vi "delete PID from engine.vi"(8 "error in (no error)":errorcluster, 9 "PID Loop in":T1, 10 "engine configuration in":refnum<class "engine configuration.lvclass">, 11 "Tagbus PID Module configuration in":refnum<class "PID Module configuration.lvclass">) -> (0 "error out":errorcluster, 1 "index":i32, 2 "engine configuration out":refnum<class "engine configuration.lvclass">, 3 "Tagbus PID Module configuration out":refnum<class "PID Module configuration.lvclass">)   [LabVIEW 2013, in "PID Module editor node.lvclass"]
uses:
  PID Module editor node.lvclass
  module/configuration/PID Module configuration.lvclass
  <vilib>/NI/Configuration Framework/serializable configuration/NISE_CEF_serializable configuration.lvclass
  <vilib>/NI/Module Execution Interface/Engine Configuration/engine configuration.lvclass
  PID array element.ctl
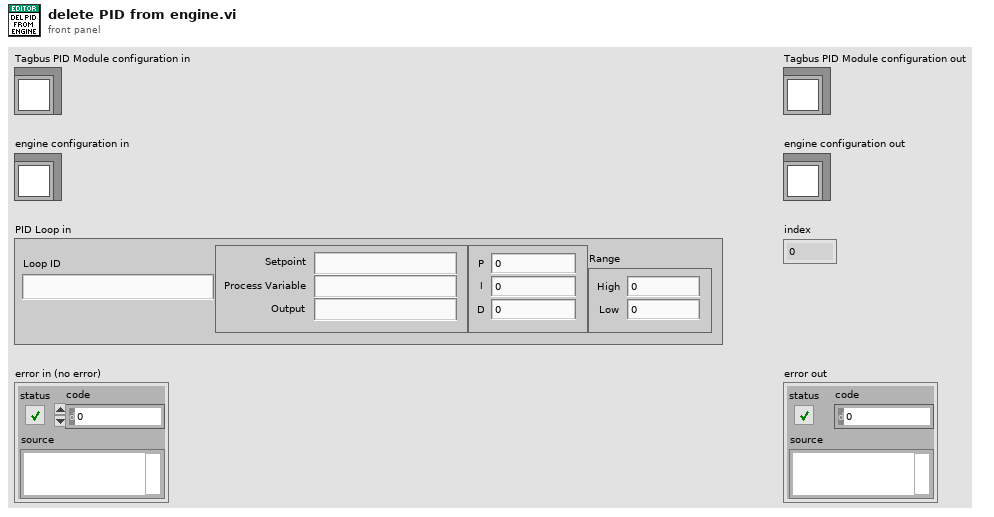
[diagram p1: front panel]
types:
  T1 = typedef "PID Module editor node.lvclass/PID array element.ctl" = cluster{"Loop ID":string, "Tags":cluster{"Setpoint":string, "Process Variable":string, "Output":string}, "Gains":cluster{"P":dbl, "I":dbl, "D":dbl}, "Range":cluster{"High":dbl, "Low":dbl}}
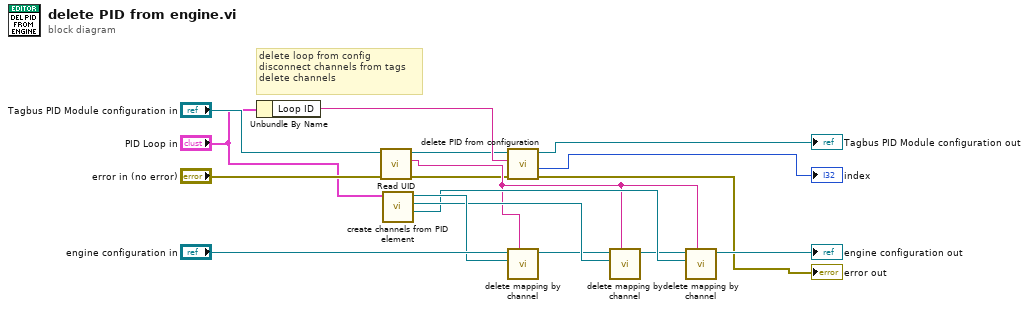
[diagram p0: block diagram]
diagram:
  # "delete loop from config\ndisconnect channels from tags\ndelete channels"
  n1 = Unbundle By Name("PID Loop in") -> ("Loop ID"=w16:string)
  n2 = call <vilib>:"Read UID.vi"("error in"="error in (no error)", "configuration in"="Tagbus PID Module configuration in") -> ("error out"=w2:errorcluster, "instance id"=w7:string, "configuration out"=w15:refnum<class "PID Module configuration.lvclass">)  [unwired: 7 in]
  n3 = call "create channels from PID element.vi"("line item in"="PID Loop in") -> ("Output Channel Out"=w8:refnum<class "TBM channel.lvclass">, "Process Variable Channel Out"=w9:refnum<class "TBM channel.lvclass">, "Setpoint Channel Out"=w10:refnum<class "TBM channel.lvclass">)  [unwired: 8 in]
  n4 = call "delete PID from configuration.vi"("error in"=w2, "PID Loop ID In"=w16, "Tagbus PID Module configuration in"=w15) -> ("error out"=→"error out":errorcluster, "index"=→"index":i32, "Tagbus PID Module configuration out"=→"Tagbus PID Module configuration out":refnum<class "PID Module configuration.lvclass">)  [unwired: 5 in, 1 out]
  n5 = call <vilib>:"delete mapping by channel.vi"("owner ID"=w7, "channel"=w10, "engine configuration in"="engine configuration in") -> ("engine configuration out"=w6:refnum<class "engine configuration.lvclass">)  [unwired: 7 in, 1 out]
  n6 = call <vilib>:"delete mapping by channel.vi"("owner ID"=w7, "channel"=w9, "engine configuration in"=w6) -> ("engine configuration out"=w5:refnum<class "engine configuration.lvclass">)  [unwired: 7 in, 1 out]
  n7 = call <vilib>:"delete mapping by channel.vi"("owner ID"=w7, "channel"=w8, "engine configuration in"=w5) -> ("engine configuration out"=→"engine configuration out":refnum<class "engine configuration.lvclass">)  [unwired: 7 in, 1 out]
